vi "fgt calibrate Pressure.vi"(8 "error in (no error)":errorcluster, 11 "pressureIndex":u32) -> (0 "error out":errorcluster)   [LabVIEW 2016, in "fgt_SDK.lvlib"]
doc: "Calibrate internal pressure depending on atmospheric pressure.\nAfter calling this function 0 pressure value corresponds to atmospheric pressure.\nDuring calibration step no pressure order is accepted. Total duration vary from 3s to 8s."
uses:
  fgt_SDK.lvlib
  dlls/fgt_SDK_32.dll
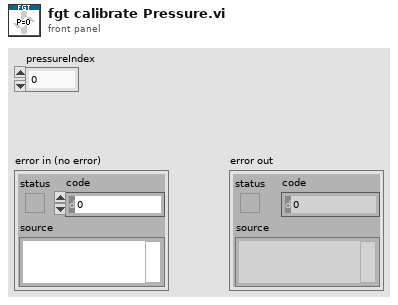
[diagram p1: front panel]
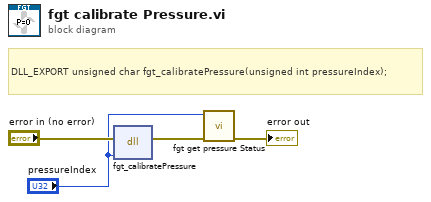
[diagram p0: block diagram]
diagram:
  # "DLL_EXPORT unsigned char fgt_calibratePressure(unsigned int pressureIndex);"
  n1 = dll-call lib="PTH2Zabs D\nMes DocumentsDéveloppementFluigentSDKsfgt-sdk-labviewdllsfgt_SDK_*.*" fn="fgt_calibratePressure"(error in="error in (no error)", "pressureIndex"="pressureIndex") -> (error out=w3:errorcluster)  [unwired: 4 in, 1 out]
  n2 = call "fgt get pressure Status.vi"("error in (no error)"=w3, "pressureIndex"="pressureIndex") -> ("error out"=→"error out":errorcluster)  [unwired: 9 in]
